vi "tdsget.vi"(1 "VISA Port In":refnum<visa-resource-name>, 7 "Channel Number":u16=1 min=1 max=2 step=1, 9 "ps/point":u32, 11 "ns/div":u32, 12 "Error In (No Error)":errorcluster) -> (3 "VISA Port Out":refnum<visa-resource-name>, 8 "TDS Data":u16[](array[numeric]), 14 "Error Out":errorcluster)   [LabVIEW 2009]
panel:
  out "Numeric":i32
  out "read buffer":string
  in  "Required TDS Data Type":u16[](array[numeric])
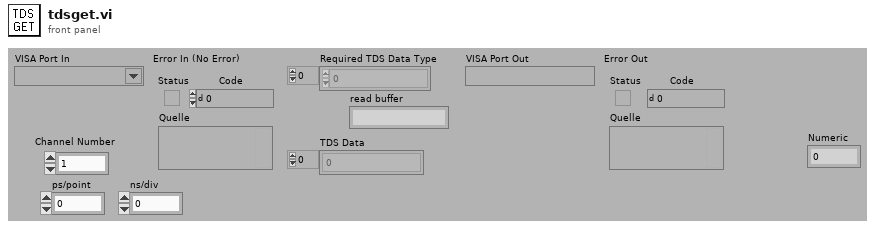
[diagram p1: front panel]
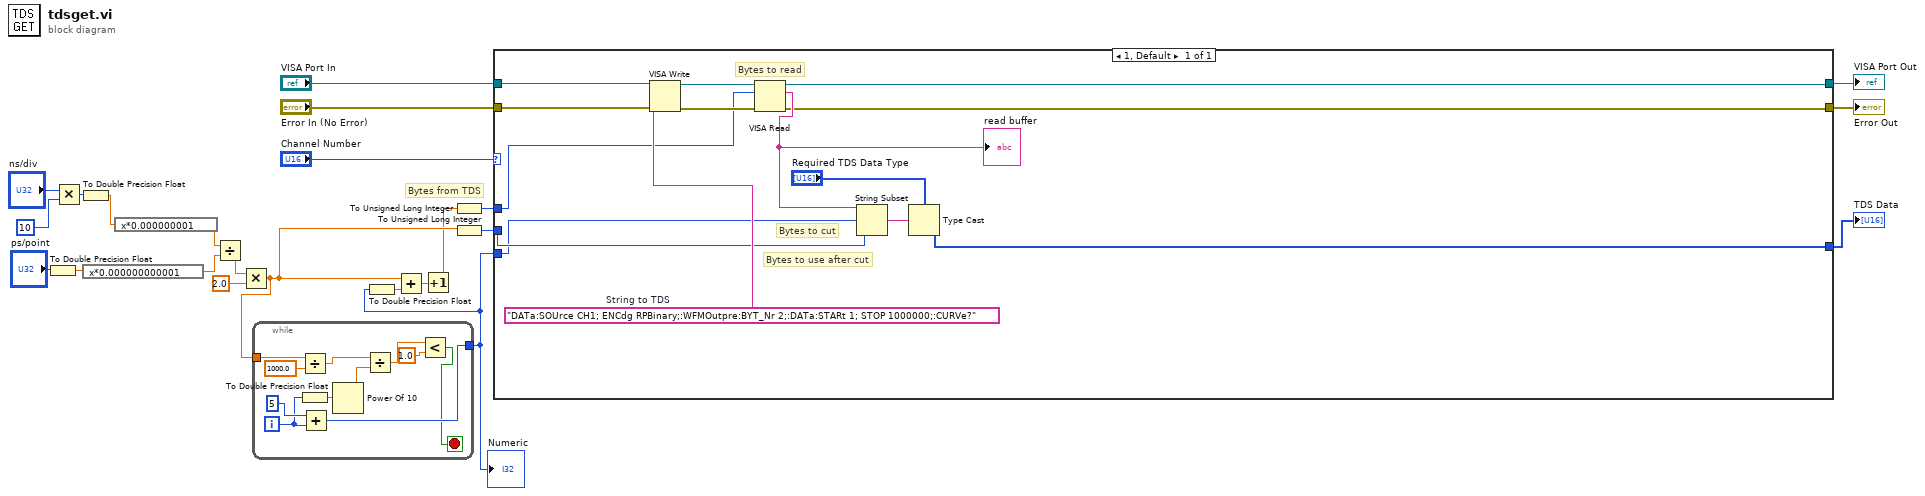
[diagram p0: block diagram]
diagram:
  # "Bytes from TDS"
  n1 = To Double Precision Float(number="ps/point") -> (double precision float=w13:dbl)
  n2 = Multiply(x="ns/div", y=u32 10) -> (x*y=w15:u32)
  n3 = To Double Precision Float(number=w15) -> (double precision float=w12:dbl)
  n4 = expression code="x*0.000000000001"(w13) -> (w10:dbl)
  n5 = expression code="x*0.000000001"(w12) -> (w11:dbl)
  n6 = Divide(x=w11, y=w10) -> (x/y=w6:dbl)
  n7 = Multiply(x=w6, y=2.0) -> (x*y=w5:dbl)
  n8 = while {
    tunnel: w5 -> [w30]
    tunnel: [w33] -> w3
    i -> [w32]
    stop <- w24 stop-if-true
    n9 = Divide(x=w30, y=1000.0) -> (x/y=w26:dbl)
    n10 = To Double Precision Float(number=w32) -> (double precision float=w31:dbl)
    n11 = Add(x=5, y=w32) -> (x+y=w33:i32)
    n12 = Power Of 10(x=w31) -> (10^x=w27:dbl)
    n13 = Divide(x=w26, y=w27) -> (x/y=w25:dbl)
    n14 = Less?(x=w25, y=1.0) -> (x < y?=w24:bool)
  }
  "Numeric" <- w3
  n15 = To Double Precision Float(number=w3) -> (double precision float=w4:dbl)
  n16 = Add(x=w5, y=w4) -> (x+y=w2:dbl)
  n17 = Increment(x=w2) -> (x+1=w1:dbl)
  n18 = To Unsigned Long Integer(number=w1) -> (unsigned 32bit integer=w8:u32)
  n19 = To Unsigned Long Integer(number=w5) -> (unsigned 32bit integer=w7:u32)
  n20 = case shown="1, Default" "Channel Number" {
    tunnel: [w39] -> w23
    tunnel: "Error In (No Error)" -> [w48]
    tunnel: "VISA Port In" -> [w47]
    tunnel: [w40] -> w20
    tunnel: [w38] -> w19
    tunnel: w8 -> [w37]
    tunnel: w7 -> [w36]
    tunnel: w3 -> [w35]
    frame 1, Default {
      w46 = "DATa:SOUrce CH1; ENCdg RPBinary;:WFMOutpre:BYT_Nr 2;:DATa:STARt 1; STOP 1000000;:CURVe?"  # String to TDS
      # "Bytes to use after cut"
      # "Bytes to cut"
      # "Bytes to read"
      n21 = VISA Write(VISA resource name=w47, write buffer=w46, error in (no error)=w48) -> (VISA resource name out=w43:refnum<visa-resource-name>, error out=w42:errorcluster)  [unwired: 1 out]
      n22 = VISA Read(VISA resource name=w43, byte count=w37, error in (no error)=w42) -> (VISA resource name out=w39:refnum<visa-resource-name>, read buffer=w41:string, error out=w38:errorcluster)  [unwired: 1 out]
      "read buffer" <- w41
      n23 = String Subset(string=w41, offset (0)=w35, length (rest)=w36) -> (substring=w44:string)
      n24 = Type Cast(type="Required TDS Data Type", x=w44) -> (*(type *) &x=w40:u16[])
    }
  }
  "Error Out" <- w19
  "VISA Port Out" <- w23
  "TDS Data" <- w20
